vi "ToNumeric.vi"(8 "error in":errorcluster, 11 "Generic":refnum<class "Generic.lvclass">) -> (0 "error out":errorcluster, 3 "Numeric out":refnum<class "Numeric.lvclass">)   [LabVIEW 2014, in "Raspberry Pi Compatible Compiler for LabVIEW.lvlib" / "Numeric.lvclass"]
uses:
  Numeric.lvclass
  Generic/Generic.lvclass
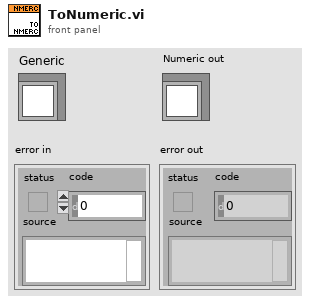
[diagram p1: front panel]
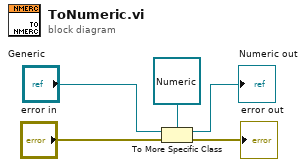
[diagram p0: block diagram]
diagram:
  n1 = To More Specific Class(target class=refnum<class "Numeric.lvclass"> refnum ("Numeric in"), reference="Generic", error in="error in") -> (specific class reference=→"Numeric out":refnum<class "Numeric.lvclass">, error out=→"error out":errorcluster)
